vi "_readNumber.vi"(8 "error in (no error)":errorcluster, 11 "tJSONParser in":refnum<class "tJSONParser.lvclass">) -> (0 "error out":errorcluster, 2 "tBSONElement Out":refnum<class "tBSONElement.lvclass">, 3 "tJSONParser out":refnum<class "tJSONParser.lvclass">)   [LabVIEW 2013, in "JSON.lvlib" / "tJSONParser.lvclass"]
doc: "Reads in a number and returns it as a tBSONElement for storage in a tBSONDocument. The number can be an integer or floating point number. Floating point numbers can also be expressed in scientific notation."
uses:
  tJSONParser.lvclass
  BSON/tBSONElement/tBSONElement.lvclass
  BSON/BSONElements/tBSONDouble/tBSONDouble.lvclass
  BSON/BSONElements/tBSON_I32/tBSON_I32.lvclass
  _error.ctl
  BSON/BSONElements/tBSONDouble/setValue.vi
  BSON/BSONElements/tBSON_I32/setValue.vi
  <vilib>/regexp/Match Regular Expression.xnode
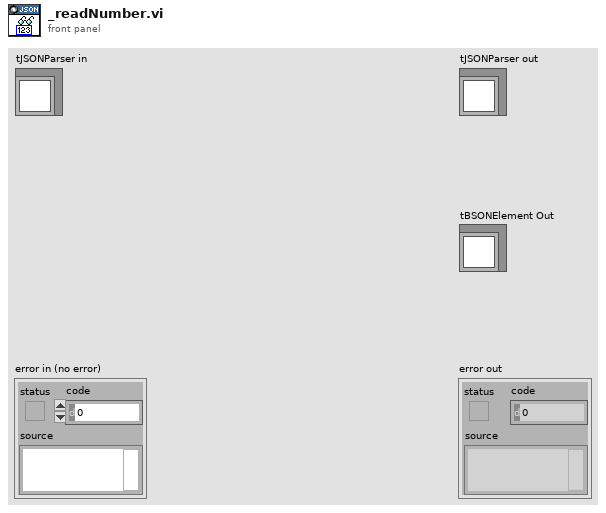
[diagram p1: front panel]
types:
  T1 = typedef "JSON.lvlib/tJSONParser.lvclass/_error.ctl" = enum16{"Missing Object Open", "Missing Pair Separator", "Missing Object End Or Separator", "Missing Pair String", "Unexpected Token", "Missing Array End Or Separator", "Invalid Escape Sequence", "Unexpected End Of File", "Invalid Unicode", "Unexpected End Of Line", "Invalid Numerical Constant"}
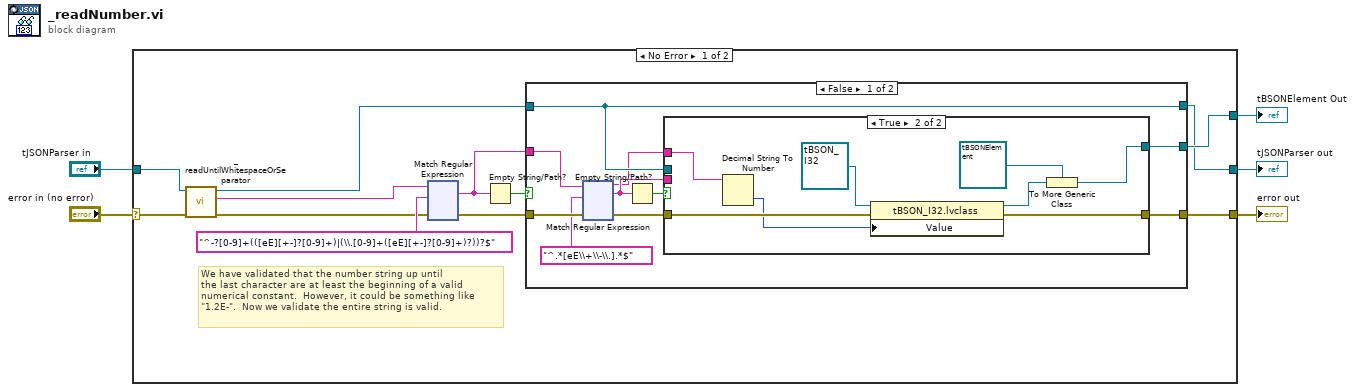
[diagram p0: block diagram]
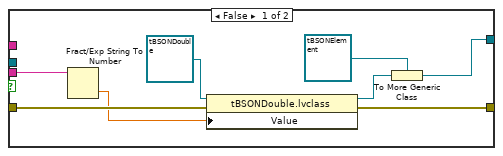
[diagram p2: hidden frame]
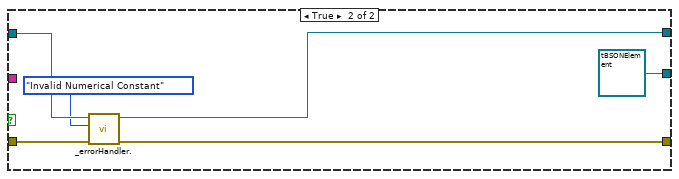
[diagram p3: hidden frame]
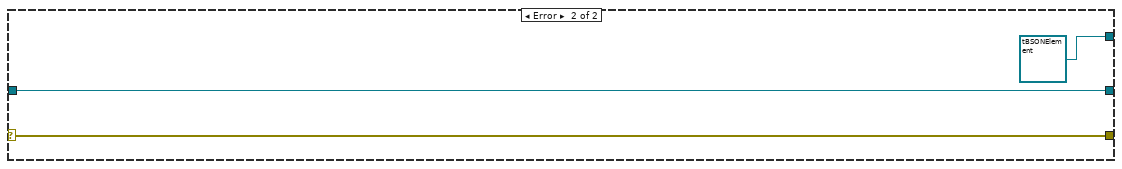
[diagram p4: hidden frame]
diagram:
  n1 = case shown="No Error" "error in (no error)" {
    selector: "error in (no error)" -> [w17 w274]
    tunnel: [w14 w274] -> w4
    tunnel: [w9 w273] -> w2
    tunnel: "tJSONParser in" -> [w16 w273]
    tunnel: [w10 refnum<class "tBSONElement.lvclass"> refnum ("tBSONElement Out")] -> w1
    frame No Error {
      # "We have validated that the number string up until\nthe last character are at least the beginning of a valid\nnumerical constant.  However, it could be something like\n\"1.2E-\".  Now we validate the entire string is valid."
      n2 = call "_readUntilWhitespaceOrSeparator.vi"("error in (no error)"=w17, "tJSONParser in"=w16) -> ("error out"=w6:errorcluster, "String Out"=w8:string, "tJSONParser out"=w7:refnum<class "tJSONParser.lvclass">)  [unwired: 7 in]
      n3 = xnode "Match Regular Expression"("input string"=w8, "regular expression"="^-?[0-9]+(([eE][+-]?[0-9]+)|(\\.[0-9]+([eE][+-]?[0-9]+)?))?$", "error in"=w6) -> ("whole match"=w11:string, "error out"=w13:errorcluster)  [unwired: 3 in, 3 out]
      n4 = Empty String/Path?(string/path=w11) -> (empty?=w12:bool)
      n5 = case shown="False" w12 {
        tunnel: [w22 w159] -> w14
        tunnel: w13 -> [w27 w160]
        tunnel: w7 -> [w20 w158]
        tunnel: w11 -> [w26 _]
        tunnel: [w21 refnum<class "tBSONElement.lvclass"> refnum ("tBSONElement Out")] -> w10
        tunnel: [w20 w156] -> w9
        frame False {
          n6 = xnode "Match Regular Expression"("input string"=w26, "regular expression"="^.*[eE\\+\\-\\.].*$", "error in"=w27) -> ("before match"=w18:string, "whole match"=w19:string, "error out"=w23:errorcluster)  [unwired: 3 in, 2 out]
          n7 = Empty String/Path?(string/path=w19) -> (empty?=w24:bool)
          n8 = case shown="True" w24 {
            tunnel: w23 -> [w30 w43]
            tunnel: [w31 w41] -> w22
            tunnel: w20 -> [_ _]
            tunnel: [w32 w39] -> w21
            tunnel: w19 -> [w29 _]
            tunnel: w18 -> [_ w36]
            frame False {
              n9 = Fract/Exp String To Number(string=w29) -> (number=w28:dbl)  [unwired: 3 in, 1 out]
              n10 = property class="tBSONDouble.lvclass"(reference=refnum<class "tBSONDouble.lvclass"> refnum ("lvMongoDriver.lvlib:BSON.lvlib:tBSONDouble.lvclass"), error in=w30, "Value"=w28) -> (reference out=w34:refnum<class "tBSONDouble.lvclass">, error out=w31:errorcluster)
              n11 = To More Generic Class(target class=refnum<class "tBSONElement.lvclass"> refnum ("tBSONElement Out"), reference=w34) -> (generic class reference=w32:refnum<class "tBSONElement.lvclass">)
            }
            frame True {
              n12 = Decimal String To Number(string=w36) -> (number=w37:i32)  [unwired: 2 in, 1 out]
              n13 = property class="tBSON_I32.lvclass"(reference=refnum<class "tBSON_I32.lvclass"> refnum ("lvMongoDriver.lvlib:BSON.lvlib:tBSON_I32.lvclass"), error in=w43, "Value"=w37) -> (reference out=w40:refnum<class "tBSON_I32.lvclass">, error out=w41:errorcluster)
              n14 = To More Generic Class(target class=refnum<class "tBSONElement.lvclass"> refnum ("tBSONElement Out"), reference=w40) -> (generic class reference=w39:refnum<class "tBSONElement.lvclass">)
            }
          }
        }
        frame True {
          n15 = call "_errorHandler..vi"("error in (no error)"=w160, "Error Type"=_error."Invalid Numerical Constant", "JSON Parser In"=w158) -> ("error out"=w159:errorcluster, "JSON Parser Out"=w156:refnum<class "tJSONParser.lvclass">)  [unwired: 7 in]
        }
      }
    }
    frame Error {
    }
  }
  "error out" <- w4
  "tJSONParser out" <- w2
  "tBSONElement Out" <- w1
